vi "Select_Waveform_By_Name_rev_160122_A.vi"(10 "Array":string[](array[string])=["HS_P_20", "HS_P_21", "HS_P_22"], 11 "Waveform Array":waveform(dbl)[](array[waveform])) -> (3 "Array 2":waveform(dbl)[](array[waveform]))   [LabVIEW 2017]
uses:
  <vilib>/Waveform/WDTOps.llb/WDT Index Channel by Name DBL.vi
panel:
  in  "Array 3":string[](array[string])=["HS_P_20", "HS_P_21", "HS_P_22"]
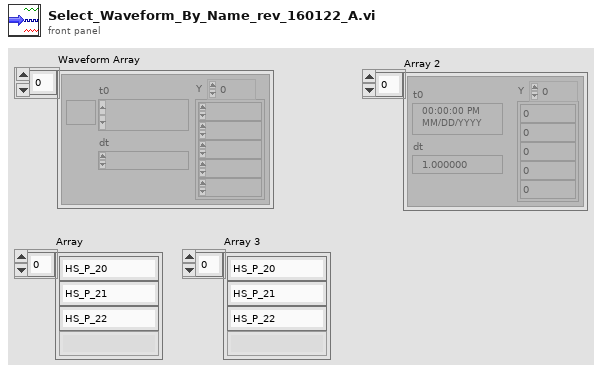
[diagram p1: front panel]
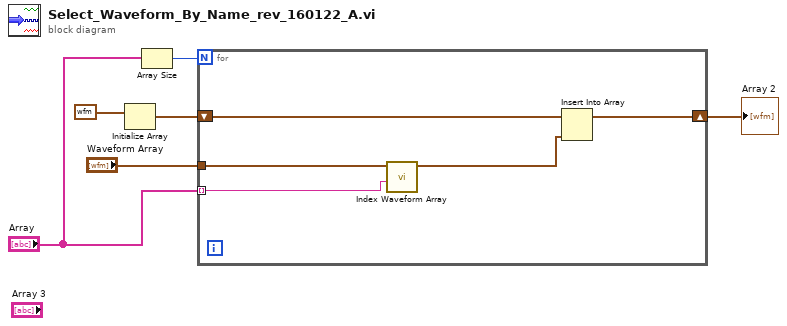
[diagram p0: block diagram]
diagram:
  n1 = Initialize Array(waveform(dbl) {"t0"=timestamp(0 s since 1904-01-01), "dt"=1.0, "Y"=[]} ("Waveform")) -> (w5:waveform(dbl)[])  [unwired: 1 in]
  n2 = Array Size(array="Array") -> (size(s)=w3:i32)
  n3 = for {
    N: w3 -> [_]
    shift-right: [w10] -> w2
    shift-left: w5 -> [w11]
    tunnel: "Waveform Array" -> [w9]
    tunnel: "Array" -> [w8] mode=indexing
    n4 = call-poly <vilib>:"Index Waveform Array.vi"("channel name"=w8, "waveform array"=w9) -> ("waveform"=w7:waveform(dbl))  [unwired: 8 in, 1 out]
    n5 = Insert Into Array(array=w11, new element=w7) -> (w10:waveform(dbl)[])  [unwired: 1 in]
  }
  "Array 2" <- w2
